vi "GateDelay_Control_V3.vi"() -> ()   [LabVIEW 2014]
uses:
  GateDelayAction_TypeDef.ctl
  <vilib>/Utility/file.llb/Read From Spreadsheet File (DBL).vi
  <vilib>/Utility/file.llb/Write To Spreadsheet File (DBL).vi
panel:
  in  "Load":bool
  in  "Save":bool
  in  "GO":bool
  in  "5":bool
  in  "4":bool
  in  "3":bool
  in  "2":bool
  in  "1":bool
  in  "0":bool
  in  "Exit":bool
  in  "Window Width (ns)":dbl(slide) min=0.0 max=9.7904 step=0.0095703125 scale=0.0..10.0
  in  "Window Delay (ns)":dbl(slide) min=0.0 max=19.9902 step=0.009765625 scale=0.0..20.0
  in  "Laser Delay (ns)":dbl(slide) min=0.0 max=19.9902 step=0.009765625 scale=0.0..20.0
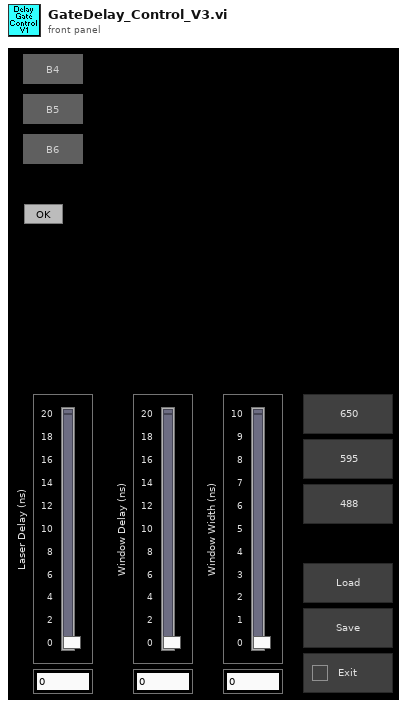
[diagram p1: front panel]
types:
  T1 = typedef "GateDelayAction_TypeDef.ctl" = enum16{"Set Laser Delay", "Set Window Delay", "Set Window Width", "Get Delays", "Exit", "CloseConnections", "Initialize"}
  T2 = enum8{"Enabled", "Disabled", "Disabled and Grayed Out"}
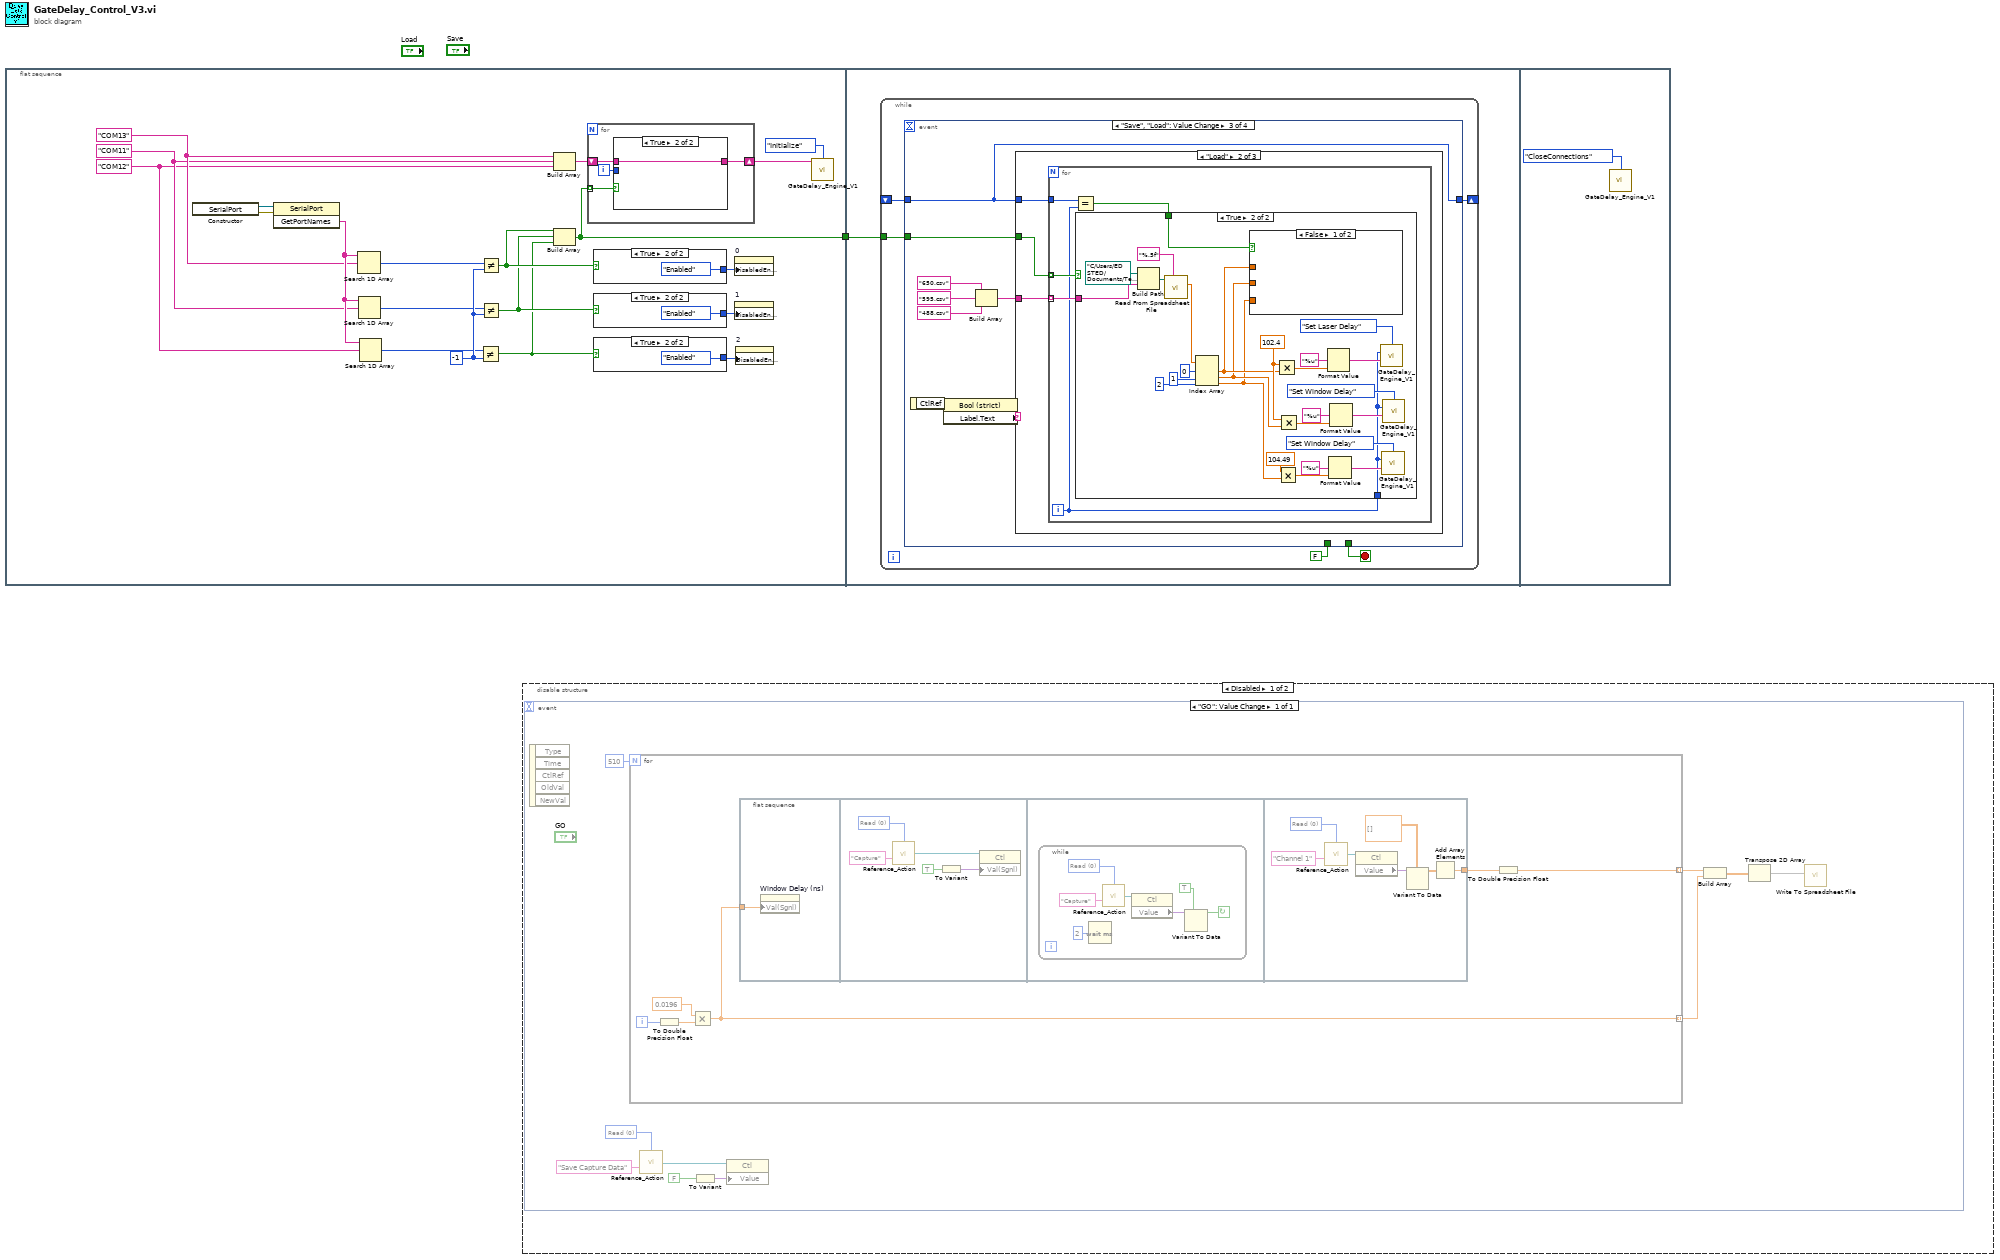
[diagram p0: block diagram]
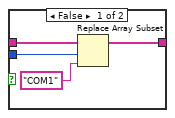
[diagram p3: hidden frame]
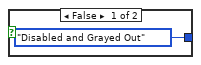
[diagram p4: hidden frame]
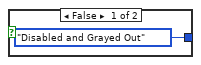
[diagram p5: hidden frame]
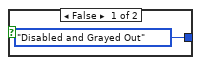
[diagram p6: hidden frame]
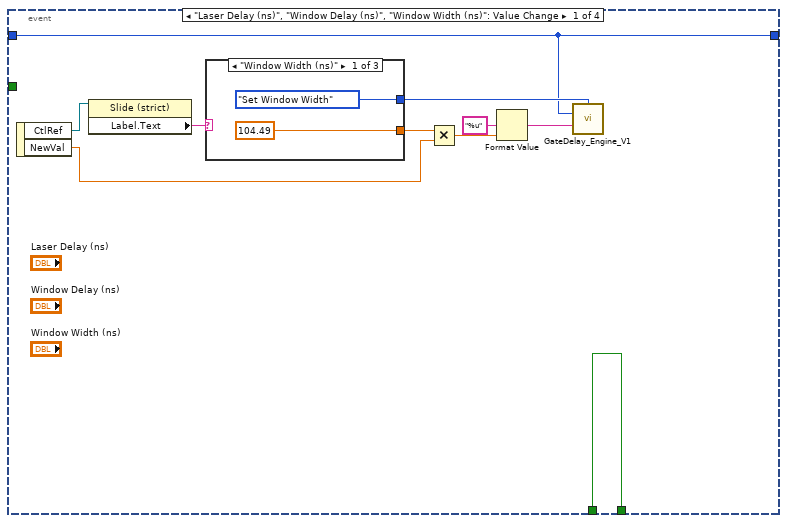
[diagram p7: hidden frame]
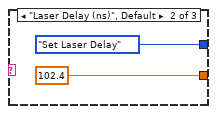
[diagram p8: hidden frame]
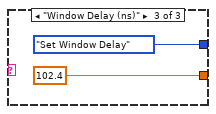
[diagram p9: hidden frame]
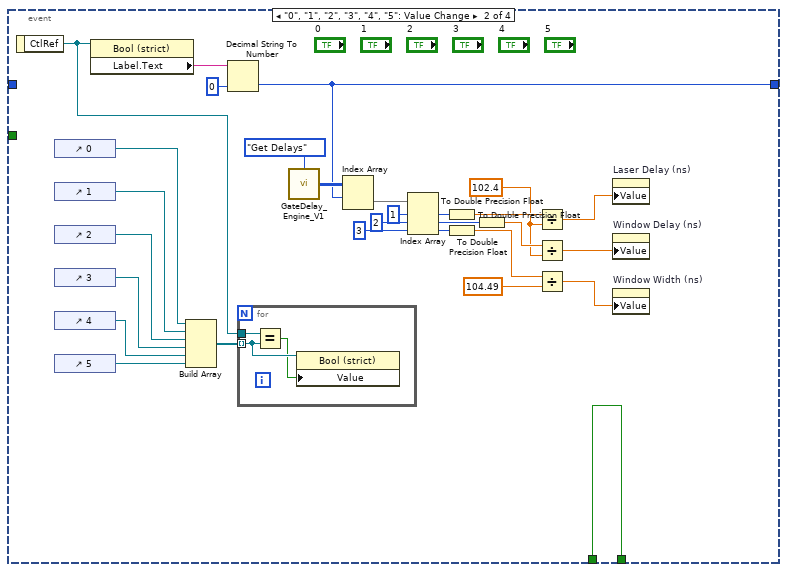
[diagram p10: hidden frame]
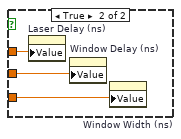
[diagram p13: hidden frame]
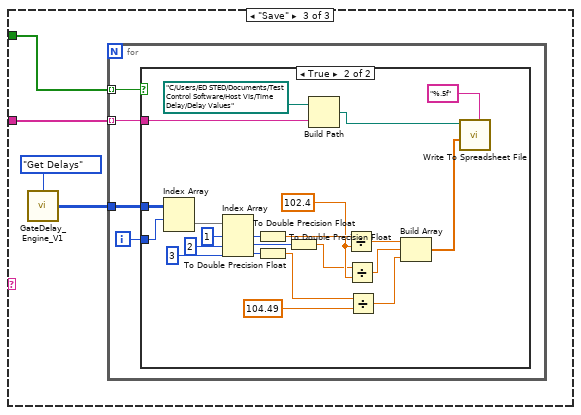
[diagram p14: hidden frame]
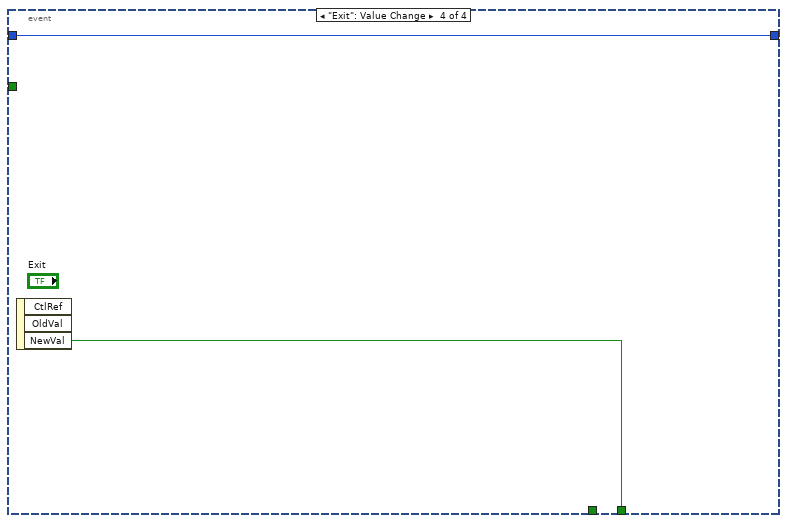
[diagram p16: hidden frame]
diagram:
  n1 = flat-sequence {
    tunnel: [w2] -> w1
    tunnel: w1 -> [w37]
    frame #0 {
      w12 = -1 ("y")
      w3 = "COM12"
      w4 = "COM11"
      w5 = "COM13"
      n2 = constructor class="SerialPort"() -> (reference out=w11:refnum<k24>, error out=w10:errorcluster)  [unwired: 3 in, 1 out]
      n3 = invoke class="SerialPort" method="GetPortNames"(reference=w11, error in=w10) -> ("GetPortNames"=w7:string[])  [unwired: 1 in, 2 out]
      n4 = Search 1D Array(1D array=w7, element=w5) -> (index of element=w9:i32)  [unwired: 1 in]
      n5 = Search 1D Array(1D array=w7, element=w4) -> (index of element=w8:i32)  [unwired: 1 in]
      n6 = Search 1D Array(1D array=w7, element=w3) -> (index of element=w6:i32)  [unwired: 1 in]
      n7 = Not Equal?(x=w6, y=w12) -> (x != y?=w15:bool)
      n8 = Not Equal?(x=w9, y=w12) -> (x != y?=w17:bool)
      n9 = Not Equal?(x=w8, y=w12) -> (x != y?=w16:bool)
      n10 = Build Array(w5, w4, w3) -> (w14:string[])
      n11 = Build Array(w17, w16, w15) -> (w2:bool[])
      n12 = for {
        tunnel: w2 -> [w25] mode=indexing
        shift-right: [w22] -> w13
        shift-left: w14 -> [w24]
        i -> [w23]
        n13 = case shown="True" w25 {
          tunnel: w24 -> [w29 w30]
          tunnel: w23 -> [w28 _]
          tunnel: [w27 w30] -> w22
          frame False {
            n14 = Replace Array Subset(array=w29, new element="COM1" ("new element/subarray"), index=w28) -> (w27:string[])
          }
          frame True {
          }
        }
      }
      n15 = case shown="True" w17 {
        tunnel: [T2."Disabled and Grayed Out" ("Disabled") T2."Enabled" ("Disabled")] -> w20
        frame False {
        }
        frame True {
        }
      }
      n16 = case shown="True" w16 {
        tunnel: [T2."Disabled and Grayed Out" ("Disabled") T2."Enabled" ("Disabled")] -> w19
        frame False {
        }
        frame True {
        }
      }
      n17 = case shown="True" w15 {
        tunnel: [T2."Disabled and Grayed Out" ("Disabled") T2."Enabled" ("Disabled")] -> w18
        frame False {
        }
        frame True {
        }
      }
      n18 = property on="0" class="Bool (strict)"("DisabledEnum"=w20) -> ()  [unwired: 2 in, 2 out]
      n19 = property on="1" class="Bool (strict)"("DisabledEnum"=w19) -> ()  [unwired: 2 in, 2 out]
      n20 = property on="2" class="Bool (strict)"("DisabledEnum"=w18) -> ()  [unwired: 2 in, 2 out]
      n21 = call "GateDelay_Engine_V1.vi"("Port Array"=w13, "DelayGate Action"=GateDelayAction_TypeDef."Initialize") -> ()  [unwired: 13 in, 1 out]
    }
    frame #1 {
      n22 = while {
        shift-right: [w40] -> _
        shift-left: _ -> [w39]
        tunnel: w37 -> [w38]
        stop <- w42 stop-if-true
        n23 = event shown="[2] \"Save\", \"Load\": Value Change" {
          selector: _ -> [_ _ _ _]
          dyn-events: _ -> [_ _ _ _]
          timeout: _ -> [_ _ _ _]
          tunnel: [w44 w87 _ w168] -> w42
          tunnel: FALSE -> [w44 w87 _ _]
          tunnel: [w43 w74 w91 w167] -> w40
          tunnel: w39 -> [w43 _ w91 w167]
          tunnel: w38 -> [_ _ w96 _]
          event "Laser Delay (ns)", "Window Delay (ns)", "Window Width (ns)": Value Change {
            n24 = event-data() -> ("CtlRef"=w52:refnum<vi>, "NewVal"=w49:dbl)  [unwired: 1 in]
            n25 = property class="Slide (strict)"(reference=w52) -> ("Label.Text"=w51:string)  [unwired: 1 in, 2 out]
            n26 = case shown="\"Window Width (ns)\"" w51 {
              tunnel: [GateDelayAction_TypeDef."Set Window Width" ("DelayGate Action") GateDelayAction_TypeDef."Set Laser Delay" ("DelayGate Action") GateDelayAction_TypeDef."Set Window Delay" ("DelayGate Action")] -> w45
              tunnel: [104.49 102.4 102.4] -> w50
              frame "Window Width (ns)" {
              }
              frame "Laser Delay (ns)", Default {
              }
              frame "Window Delay (ns)" {
              }
            }
            n27 = Multiply(x=w50, y=w49) -> (x*y=w48:dbl)
            n28 = Format Value(format string="%u", value (0)=w48) -> (output string=w46:string)  [unwired: 1 in]
            n29 = call "GateDelay_Engine_V1.vi"("DelayGate Action"=w45, "Device Index"=w43, "Delay Value (steps)"=w46) -> ()  [unwired: 12 in, 1 out]
          }
          event "0", "1", "2", "3", "4", "5": Value Change {
            w62 = 102.4
            n30 = event-data() -> ("CtlRef"=w77:refnum<vi>)  [unwired: 1 in]
            n31 = control-ref of="0"() -> (w84:refnum<vi>)
            n32 = control-ref of="1"() -> (w83:refnum<vi>)
            n33 = control-ref of="2"() -> (w82:refnum<vi>)
            n34 = control-ref of="3"() -> (w81:refnum<vi>)
            n35 = control-ref of="4"() -> (w80:refnum<vi>)
            n36 = control-ref of="5"() -> (w79:refnum<vi>)
            n37 = property class="Bool (strict)"(reference=w77) -> ("Label.Text"=w86:string)  [unwired: 1 in, 2 out]
            n38 = Build Array(w84, w83, w82, w81, w80, w79) -> (w78:refnum<vi>[])
            n39 = Decimal String To Number(string=w86, default (0L)=0 ("default (0 I32)")) -> (number=w74:i32)  [unwired: 1 in, 1 out]
            n40 = for {
              tunnel: w78 -> [w89] mode=indexing
              tunnel: w77 -> [w90]
              n41 = Equal?(x=w90, y=w89) -> (x = y?=w88:bool)
              n42 = property class="Bool (strict)"(reference=w89, "Value"=w88) -> ()  [unwired: 1 in, 2 out]
            }
            n43 = call "GateDelay_Engine_V1.vi"("DelayGate Action"=GateDelayAction_TypeDef."Get Delays") -> ("Current Delays"=w75:i32[][])  [unwired: 14 in]
            n44 = Index Array(array=w75, index (row)=w74) -> (element=w73:i32[])  [unwired: 1 in]
            n45 = Index Array(array=w73, index #1=1 ("index"), index #2=2 ("index"), index #3=3 ("index")) -> (element #1=w69:i32, element #2=w68:i32, element #3=w67:i32)
            n46 = To Double Precision Float(number=w69) -> (double precision float=w66:dbl)
            n47 = To Double Precision Float(number=w67) -> (double precision float=w64:dbl)
            n48 = To Double Precision Float(number=w68) -> (double precision float=w65:dbl)
            n49 = Divide(x=w66, y=w62) -> (x/y=w59:dbl)
            n50 = Divide(x=w65, y=w62) -> (x/y=w61:dbl)
            n51 = Divide(x=w64, y=104.49) -> (x/y=w60:dbl)
            n52 = property on="Laser Delay (ns)" class="Slide (strict)"("Value"=w59) -> ()  [unwired: 2 in, 2 out]
            n53 = property on="Window Delay (ns)" class="Slide (strict)"("Value"=w61) -> ()  [unwired: 2 in, 2 out]
            n54 = property on="Window Width (ns)" class="Slide (strict)"("Value"=w60) -> ()  [unwired: 2 in, 2 out]
          }
          event "Save", "Load": Value Change {
            n55 = event-data() -> ("CtlRef"=w98:refnum<vi>)  [unwired: 1 in]
            n56 = property class="Bool (strict)"(reference=w98) -> ("Label.Text"=w97:string)  [unwired: 1 in, 2 out]
            n57 = Build Array("650.csv", "595.csv", "488.csv") -> (w92:string[])
            n58 = case shown="\"Load\"" w97 {
              tunnel: w96 -> [_ w101 w139]
              tunnel: w92 -> [_ w100 w137]
              tunnel: w91 -> [_ w99 _]
              frame "", Default {
              }
              frame "Load" {
                n59 = for {
                  tunnel: w101 -> [w106] mode=indexing
                  tunnel: w100 -> [w105] mode=indexing
                  tunnel: w99 -> [w103]
                  i -> [w102]
                  n60 = Equal?(x=w103, y=w102) -> (x = y?=w104:bool)
                  n61 = case shown="True" w106 {
                    tunnel: w105 -> [_ w132]
                    tunnel: w102 -> [_ w111]
                    tunnel: w104 -> [_ w110]
                    frame False {
                    }
                    frame True {
                      w117 = 102.4 ("x")
                      n62 = Build Path(base path=path "C:/Users/ED STED/Documents/Test Control Software/Host VIs/Time Delay/Delay Values", name or relative path=w132) -> (appended path=w130:path)
                      n63 = call-poly <vilib>:"Read From Spreadsheet File.vi"("format (%.3f)"="%.5f", "file path (dialog if empty)"=w130) -> ("first row"=w129:dbl[])  [unwired: 5 in, 4 out]
                      n64 = Index Array(array=w129, index #1=0 ("index"), index #2=1 ("index"), index #3=2 ("index")) -> (element #1=w109:dbl, element #2=w108:dbl, element #3=w107:dbl)
                      n65 = case shown="False" w110 {
                        tunnel: w109 -> [_ w134]
                        tunnel: w108 -> [_ w135]
                        tunnel: w107 -> [_ w136]
                        frame False {
                        }
                        frame True {
                          n66 = property on="Laser Delay (ns)" class="Slide (strict)"("Value"=w134) -> ()  [unwired: 2 in, 2 out]
                          n67 = property on="Window Delay (ns)" class="Slide (strict)"("Value"=w135) -> ()  [unwired: 2 in, 2 out]
                          n68 = property on="Window Width (ns)" class="Slide (strict)"("Value"=w136) -> ()  [unwired: 2 in, 2 out]
                        }
                      }
                      n69 = Multiply(x=w117, y=w109) -> (x*y=w125:dbl)
                      n70 = Multiply(x=104.49, y=w107) -> (x*y=w116:dbl)
                      n71 = Multiply(x=w117, y=w108) -> (x*y=w118:dbl)
                      n72 = Format Value(format string="%u", value (0)=w125) -> (output string=w123:string)  [unwired: 1 in]
                      n73 = Format Value(format string="%u", value (0)=w116) -> (output string=w114:string)  [unwired: 1 in]
                      n74 = Format Value(format string="%u", value (0)=w118) -> (output string=w120:string)  [unwired: 1 in]
                      n75 = call "GateDelay_Engine_V1.vi"("DelayGate Action"=GateDelayAction_TypeDef."Set Laser Delay", "Device Index"=w111, "Delay Value (steps)"=w123) -> ()  [unwired: 12 in, 1 out]
                      n76 = call "GateDelay_Engine_V1.vi"("DelayGate Action"=GateDelayAction_TypeDef."Set Window Delay", "Device Index"=w111, "Delay Value (steps)"=w114) -> ()  [unwired: 12 in, 1 out]
                      n77 = call "GateDelay_Engine_V1.vi"("DelayGate Action"=GateDelayAction_TypeDef."Set Window Delay", "Device Index"=w111, "Delay Value (steps)"=w120) -> ()  [unwired: 12 in, 1 out]
                    }
                  }
                }
              }
              frame "Save" {
                n78 = call "GateDelay_Engine_V1.vi"("DelayGate Action"=GateDelayAction_TypeDef."Get Delays") -> ("Current Delays"=w138:i32[][])  [unwired: 14 in]
                n79 = for {
                  tunnel: w139 -> [w144] mode=indexing
                  tunnel: w138 -> [w143]
                  tunnel: w137 -> [w141] mode=indexing
                  i -> [w142]
                  n80 = case shown="True" w144 {
                    tunnel: w143 -> [_ w166]
                    tunnel: w142 -> [_ w165]
                    tunnel: w141 -> [_ w148]
                    frame False {
                    }
                    frame True {
                      w156 = 102.4
                      n81 = Index Array(array=w166, index (row)=w165) -> (element=w164:i32[])  [unwired: 1 in]
                      n82 = Index Array(array=w164, index #1=1 ("index"), index #2=2 ("index"), index #3=3 ("index")) -> (element #1=w160:i32, element #2=w159:i32, element #3=w158:i32)
                      n83 = To Double Precision Float(number=w160) -> (double precision float=w157:dbl)
                      n84 = To Double Precision Float(number=w158) -> (double precision float=w154:dbl)
                      n85 = To Double Precision Float(number=w159) -> (double precision float=w155:dbl)
                      n86 = Build Path(base path=path "C:/Users/ED STED/Documents/Test Control Software/Host VIs/Time Delay/Delay Values", name or relative path=w148) -> (appended path=w145:path)
                      n87 = Divide(x=w157, y=w156) -> (x/y=w152:dbl)
                      n88 = Divide(x=w155, y=w156) -> (x/y=w151:dbl)
                      n89 = Divide(x=w154, y=104.49) -> (x/y=w150:dbl)
                      n90 = Build Array(w152, w151, w150) -> (w149:dbl[])
                      n91 = call-poly <vilib>:"Write To Spreadsheet File.vi"("format (%.3f)"="%.5f", "1D data"=w149, "file path (dialog if empty)"=w145) -> ()  [unwired: 5 in, 1 out]
                    }
                  }
                }
              }
            }
          }
          event "Exit": Value Change {
            n92 = event-data() -> ("NewVal"=w168:bool)  [unwired: 1 in, 2 out]
          }
        }
      }
    }
    frame #2 {
      n93 = call "GateDelay_Engine_V1.vi"("DelayGate Action"=GateDelayAction_TypeDef."CloseConnections") -> ()  [unwired: 14 in, 1 out]
    }
  }
  n94 = disable-structure shown="Disabled" {
    frame Disabled {
      n95 = event shown="[0] \"GO\": Value Change" {
        selector: _ -> [_]
        dyn-events: _ -> [_]
        timeout: _ -> [_]
        event "GO": Value Change {
          w175 = u16 0 items=["Read", "Initialize"] ("Action")
          n96 = event-data() -> ()  [unwired: 1 in, 5 out]
          n97 = for {
            N: 510 -> [_]
            tunnel: [w182] -> w172 mode=indexing
            tunnel: [w180] -> w173 mode=indexing
            i -> [w185]
            n98 = To Double Precision Float(number=w185) -> (double precision float=w184:dbl)
            n99 = Multiply(x=0.0196, y=w184) -> (x*y=w182:dbl)
            n100 = flat-sequence {
              tunnel: w182 -> [w186]
              tunnel: [w199] -> w181
              frame #0 {
                n101 = property on="Window Delay (ns)" class="Slide (strict)"("Val(Sgnl)"=w186) -> ()  [unwired: 2 in, 2 out]
              }
              frame #1 {
                w191 = u16 0 items=["Read", "Initialize"] ("Action")
                n102 = call "Reference_Action.vi"("Action"=w191, "Control Name"="Capture") -> ("Ref OUT"=w189:refnum<vi>)  [unwired: 12 in, 1 out]
                n103 = To Variant(anything=TRUE) -> (Variant=w187:variant)
                n104 = property class="Ctl"(reference=w189, "Val(Sgnl)"=w187) -> ()  [unwired: 1 in, 2 out]
              }
              frame #2 {
                n105 = while {
                  stop <- w193 continue-if-true
                  w196 = u16 0 items=["Read", "Initialize"] ("Action")
                  n106 = Wait (ms)(milliseconds to wait=u32 2) -> ()  [unwired: 1 out]
                  n107 = call "Reference_Action.vi"("Action"=w196, "Control Name"="Capture") -> ("Ref OUT"=w198:refnum<vi>)  [unwired: 12 in, 1 out]
                  n108 = property class="Ctl"(reference=w198) -> ("Value"=w195:variant)  [unwired: 1 in, 2 out]
                  n109 = Variant To Data(type=TRUE, Variant=w195) -> (data=w193:bool)  [unwired: 1 in, 1 out]
                }
              }
              frame #3 {
                w204 = u16 0 items=["Read", "Initialize"] ("Action")
                n110 = call "Reference_Action.vi"("Action"=w204, "Control Name"="Channel 1") -> ("Ref OUT"=w203:refnum<vi>)  [unwired: 12 in, 1 out]
                n111 = property class="Ctl"(reference=w203) -> ("Value"=w202:variant)  [unwired: 1 in, 2 out]
                n112 = Variant To Data(type=sgl[][] [], Variant=w202) -> (data=w200:sgl[][])  [unwired: 1 in, 1 out]
                n113 = Add Array Elements(numeric array=w200) -> (sum=w199:sgl)
              }
            }
            n114 = To Double Precision Float(number=w181) -> (double precision float=w180:dbl)
          }
          n115 = call "Reference_Action.vi"("Action"=w175, "Control Name"="Save Capture Data") -> ("Ref OUT"=w176:refnum<vi>)  [unwired: 12 in, 1 out]
          n116 = To Variant(anything=FALSE) -> (Variant=w177:variant)
          n117 = property class="Ctl"(reference=w176, "Value"=w177) -> ()  [unwired: 1 in, 2 out]
          n118 = Build Array(w173, w172) -> (w171:dbl[][])
          n119 = Transpose 2D Array(2D array=w171) -> (transposed array=w170:dbl[][])
          n120 = call-poly <vilib>:"Write To Spreadsheet File.vi"("2D data"=w170) -> ()  [unwired: 7 in, 1 out]
        }
      }
    }
    frame Enabled {
    }
  }
